vi "Fax.vi"(11 "IMachine In":refnum<class "IMachine.lvclass">) -> (3 "IMachine Out":refnum<class "IMachine.lvclass">)   [LabVIEW 2018, in "IMachine.lvclass"]
uses:
  IMachine.lvclass
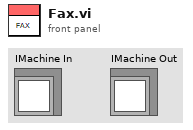
[diagram p1: front panel]
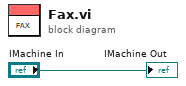
[diagram p0: block diagram]
diagram:
  "IMachine Out" <- "IMachine In"
